vi "Read Buffer.vi"(8 "error in (no error)":errorcluster, 9 "timeout ms (25000)":i32 format="%d ms", 11 "queue data in":T1={"server ID"=refnum, "Buffer data"={"decimation"=0, "avg bandwidth"=0.0, "channels"=[], "byte order"=enum."little-endian", "buffer descriptor"={"buffer type"=enum."Engine", "plugin id"=0, "group id"=0, "transfer id"=0, "offset"=0, "length"=0}, "values channels"={"index"=0, "count"=0, "engine offset"=0}, "select start offset"=18446744073709551615, "select end offset"=0, "channel index"=-1}} {"Buffer data"."channels"."configuration"."string offset" format="%d bytes"; "Buffer data"."avg bandwidth" format="%.0g bytes"}) -> (0 "error out":errorcluster, 1 "buffer data":string, 2 "values string":string, 3 "queue data out":T1={"server ID"=refnum, "Buffer data"={"decimation"=0, "avg bandwidth"=0.0, "channels"=[], "byte order"=enum."little-endian", "buffer descriptor"={"buffer type"=enum."Engine", "plugin id"=0, "group id"=0, "transfer id"=0, "offset"=0, "length"=0}, "values channels"={"index"=0, "count"=0, "engine offset"=0}, "select start offset"=18446744073709551615, "select end offset"=0, "channel index"=-1}} {"Buffer data"."channels"."configuration"."string offset" format="%d bytes"; "Buffer data"."avg bandwidth" format="%.0g bytes"}, 4 "timed out?":bool, 5 "buffer size":u64, 7 "metrics":T11)   [LabVIEW 2017, in "Data Viewer.lvlib"]
uses:
  Core/VIs/Data Viewer/Source/Data Viewer.lvlib
  Queue Data.ctl
  Buffer Data.ctl
  Core/Classes/Configuration/Core/Transfer/Channel Configuration.ctl
  Core/Typedefs/Core Channel Configuration.ctl
  Core/Typedefs/DSF Data Type.ctl
  Core/Typedefs/DSF Settings Info.ctl
  Core/Typedefs/DSF Byte Order.ctl
  Core/Classes/Thread/Data Server/DSF Buffer Subset Descriptor.ctl
  Core/Typedefs/DSF Buffer Type.ctl
  Main VI/Values Channels.ctl
  Core/Classes/Thread/Data Server/DSF Performance Metrics.ctl
  Core/DSF Core.lvlib
  Core/Classes/Configuration/Core/Channel/Channel Configuration.lvclass
  Core/Classes/Configuration/Core/Transfer/Transfer Configuration.lvclass
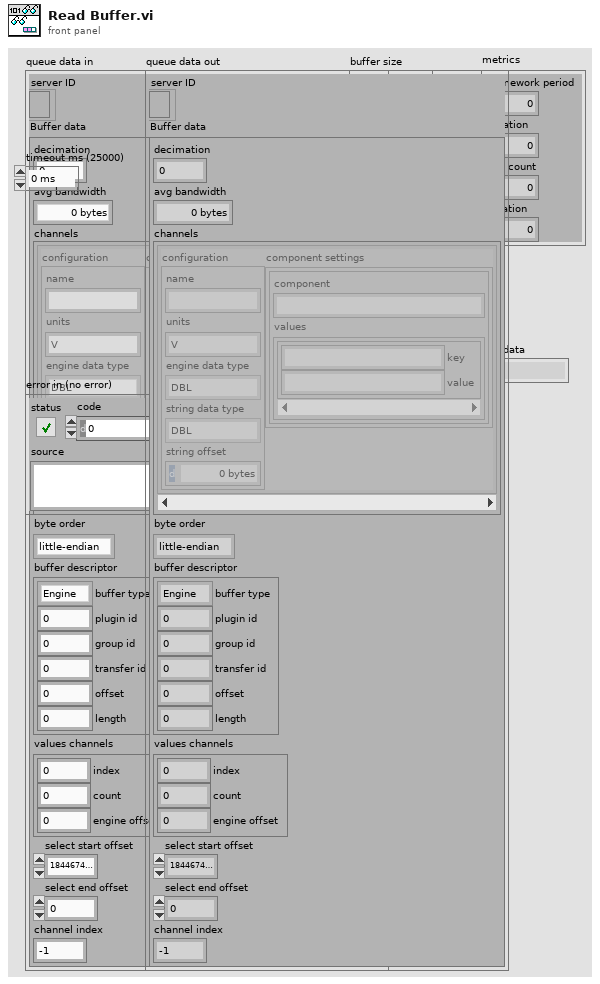
[diagram p1: front panel]
types:
  T1 = typedef "Data Viewer.lvlib/Queue Data.ctl" = cluster{"server ID":refnum<k5>, "Buffer data":T2}
  T2 = typedef "Data Viewer.lvlib/Buffer Data.ctl" = cluster{"decimation":u64, "avg bandwidth":dbl, "channels":T3[], "byte order":T7, "buffer descriptor":T8, "values channels":T10, "select start offset":u64, "select end offset":u64, "channel index":i32}
  T3 = typedef "DSF Core.lvlib/Transfer Configuration.lvclass/Channel Configuration.ctl" = cluster{"configuration":T4, "component settings":T6[]}
  T4 = typedef "DSF Core.lvlib/Channel Configuration.lvclass/Core Channel Configuration.ctl" = cluster{"name":string, "units":string, "engine data type":T5, "string data type":T5, "string offset":u64}
  T5 = typedef "DSF Core.lvlib/DSF Data Type.ctl" = enum8{"Bool", "SGL", "DBL", "I8", "I16", "I32", "I64", "U8", "U16", "U32", "U64"}
  T6 = typedef "DSF Core.lvlib/DSF Settings Info.ctl" = cluster{"component":string, "values":cluster{"key":string, "value":string}[]}
  T7 = typedef "DSF Core.lvlib/DSF Byte Order.ctl" = enum8{"big-endian", "little-endian"}
  T8 = typedef "DSF Core.lvlib/DSF Buffer Subset Descriptor.ctl" = cluster{"buffer type":T9, "plugin id":i32, "group id":i32, "transfer id":i32, "offset":u64, "length":i64}
  T9 = typedef "DSF Core.lvlib/DSF Buffer Type.ctl" = enum16{"Engine", "String"}
  T10 = typedef "Data Viewer.lvlib/Values Channels.ctl" = cluster{"index":i32, "count":i32, "engine offset":u64}
  T11 = typedef "DSF Core.lvlib/DSF Performance Metrics.ctl" = cluster{"framework period":u32, "iteration":u64, "late count":u64, "duration":u64}
  T12 = cluster{"buffer type":bool, "plugin id":bool, "group id":bool, "transfer id":bool, "offset":bool, "length":bool}
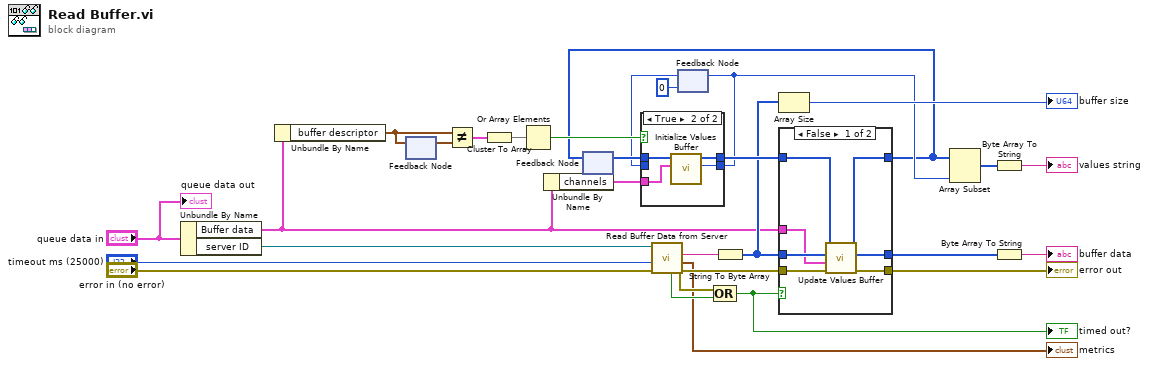
[diagram p0: block diagram]
diagram:
  n1 = Unbundle By Name("queue data in") -> ("Buffer data"=w8:T2, "server ID"=w27:refnum<k5>)
  n2 = Unbundle By Name(w8) -> ("buffer descriptor"=w6:T8)
  n3 = feedback-in #1(w6) -> ()
  n4 = feedback #1() -> (w7:T8)  [unwired: 1 in]
  n5 = Not Equal?(x=w6, y=w7) -> (x != y?=w5:T12)
  n6 = Cluster To Array(cluster=w5) -> (array=w4:bool[])
  n7 = Or Array Elements(Boolean array=w4) -> (logical OR=w3:bool)
  n8 = Unbundle By Name(w8) -> ("channels"=w14:T3[])
  n9 = feedback #2() -> (w18:u8[])  [unwired: 1 in]
  n10 = call "Read Buffer Data from Server.vi"("error in (no error)"="error in (no error)", "timeout ms (25000)"="timeout ms (25000)", "server ID in"=w27) -> ("error out"=w22:errorcluster, "metrics"=→"metrics":T11, "buffer data"=w25:string, "timed out?"=w23:bool)  [unwired: 4 in, 1 out]
  n11 = feedback #3(0 ("size")) -> (w1:i32)
  n12 = case shown="True" w3 {
    tunnel: [w31 w32] -> w19
    tunnel: w18 -> [w31 w33]
    tunnel: [w30 w35] -> w11
    tunnel: w1 -> [w30 _]
    tunnel: w14 -> [_ w34]
    frame False {
    }
    frame True {
      n13 = call "Initialize Values Buffer.vi"("channels"=w34, "values buffer in"=w33) -> ("size"=w35:i32, "values buffer out"=w32:u8[])  [unwired: 8 in]
    }
  }
  n14 = feedback-in #3(w11) -> ()
  n15 = Compound Arithmetic op=OR(w22, w23) -> (w12:bool)
  "timed out?" <- w12
  n16 = String To Byte Array(string=w25) -> (unsigned byte array=w13:u8[])
  n17 = Array Size(array=w13) -> (size(s)=→"buffer size":i32)
  n18 = case shown="False" w12 {
    tunnel: [w40 w44] -> w29
    tunnel: [w36 _] -> w9
    tunnel: w8 -> [w39 _]
    tunnel: w22 -> [w42 w44]
    tunnel: w13 -> [w41 _]
    tunnel: w19 -> [w37 w43]
    tunnel: [w38 w43] -> w2
    frame False {
      n19 = call "Update Values Buffer.vi"("error in (no error)"=w42, "buffer data"=w39, "buffer in"=w41, "values buffer in"=w37) -> ("error out"=w40:errorcluster, "buffer out"=w36:u8[], "values buffer out"=w38:u8[])  [unwired: 5 in]
    }
    frame True {
    }
  }
  "error out" <- w29
  n20 = feedback-in #2(w2) -> ()
  n21 = Array Subset(array=w2, length=w11) -> (w17:u8[])  [unwired: 1 in]
  n22 = Byte Array To String(unsigned byte array=w17) -> (string=→"values string":string)
  n23 = Byte Array To String(unsigned byte array=w9) -> (string=→"buffer data":string)
  "queue data out" <- "queue data in"
